vi "Get Singleton and Cloneable Refs.vi"(8 "error in":errorcluster) -> (0 "error out":errorcluster, 1 "Cloneable?":bool[](array[boolean]), 2 "Modules List":string[](array[string]), 3 "DQMH Modules":refnum<vi>[](array[refnum]))   [LabVIEW 2020, in "DQMH_API.lvlib"]
doc: "Gets the Singleton and Cloneable references and creates a list of each type of DQMH Modules"
uses:
  DQMH_API.lvlib
  <vilib>/Delacor/Delacor QMH/Libraries/Scripting API/DQMH_Scripting API.lvlib
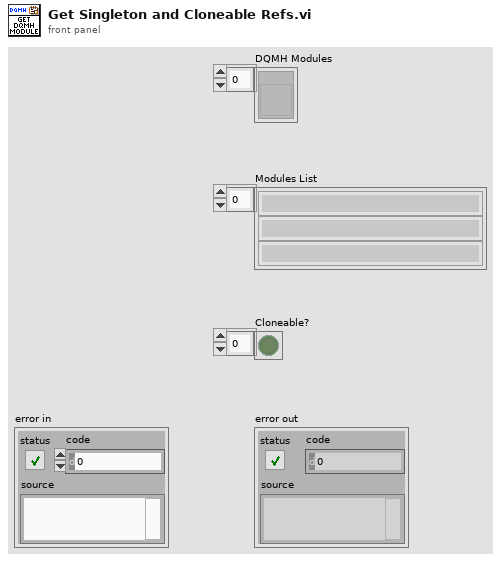
[diagram p1: front panel]
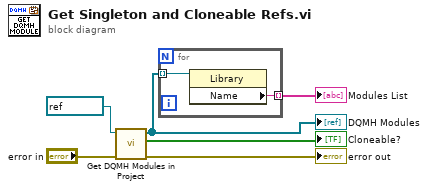
[diagram p0: block diagram]
diagram:
  n1 = call <vilib>:"Get DQMH Modules in Project.vi"("error in"="error in", "Project"=refnum<vi> refnum) -> ("error out"=→"error out":errorcluster, "Cloneable?"=→"Cloneable?":bool[], "DQMH Module Libraries"=w1:refnum<vi>[])  [unwired: 7 in]
  "DQMH Modules" <- w1
  n2 = for {
    tunnel: [w8] -> w3 mode=indexing
    tunnel: w1 -> [w7] mode=indexing
    n3 = property class="Library"(reference=w7) -> ("Name"=w8:string)  [unwired: 1 in, 2 out]
  }
  "Modules List" <- w3
